vi "PV_Gnl_WaitForViClose.vi"(8 "error in":errorcluster, 10 "TimeOut (ms)":i32, 11 "ViRefNum":refnum<vi>) -> (0 "error out":errorcluster, 3 "ViRefNumDuplicated":refnum<vi>)   [LabVIEW 2020]
doc: "Fonction :\n\nAttend si le VI entré en référence est déchargé de la mémoire, ou si le temps impartit est dépassé.\n\n*****\n\nEntrées :\n\nVIRefNum : référence du VI à vérifier. Dupliquée dans tous les cas. Cette connexion est nécessaire.\n\nTimeOut : temps impartit à cette fonction pour vérifier si le VI est déchargé de la mémoire. Cette connexion est nécessaire.\n\nerror in : entrée d'erreur.\n\n*****\n\nSorties :\n\nVIRefNumDuplicated : référence du VI.\n\nerror out : sortie d'erreur."
panel:
  # "Input"
  # "Output"
  # "Local"
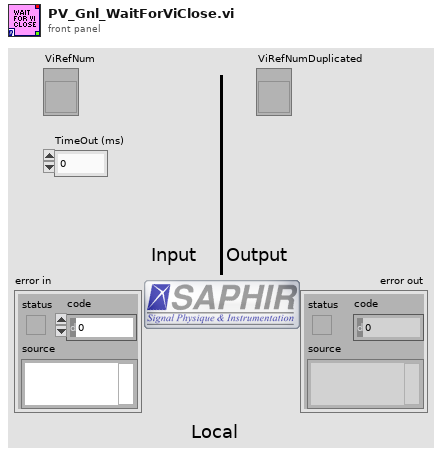
[diagram p1: front panel]
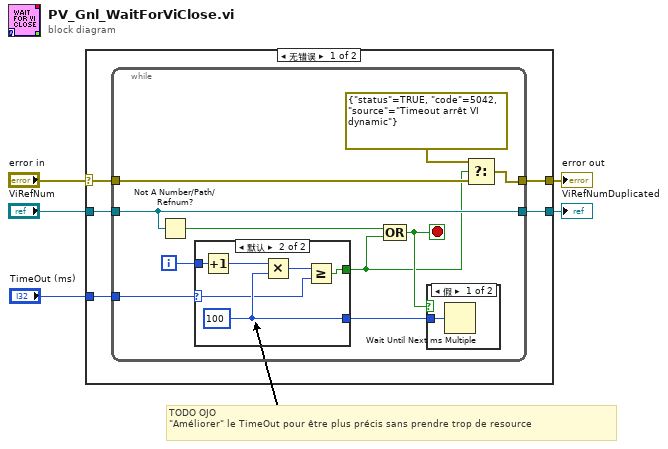
[diagram p0: block diagram]
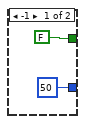
[diagram p2: hidden frame]
diagram:
  # "TODO OJO\n\"Améliorer\" le TimeOut pour être plus précis sans prendre trop de resource"
  n1 = case shown="无错误" "error in" {
    selector: "error in" -> [w9 w31]
    tunnel: [w8 w31] -> w3
    tunnel: "ViRefNum" -> [w10 w30]
    tunnel: [w7 w30] -> w4
    tunnel: "TimeOut (ms)" -> [w6 _]
    frame No Error {
      n2 = while {
        tunnel: w9 -> [w18]
        tunnel: [w20] -> w8
        tunnel: w10 -> [w16]
        tunnel: [w16] -> w7
        tunnel: w6 -> [w13]
        i -> [w14]
        stop <- w15 stop-if-true
        n3 = Not A Number/Path/Refnum?(number/path/refnum=w16) -> (NaN/Path/Refnum?=w17:bool)
        n4 = case shown="默认" w13 {
          selector: w13 -> [_ w23]
          tunnel: w14 -> [_ w25]
          tunnel: [FALSE w28] -> w11
          tunnel: [u32 50 ("millisecond multiple") w27] -> w12
          frame -1 {
          }
          frame Default {
            w27 = 100 ("y")
            n5 = Increment(x=w25) -> (x+1=w26:i32)
            n6 = Multiply(x=w26, y=w27) -> (x*y=w24:i32)
            n7 = Greater Or Equal?(x=w24, y=w23) -> (x >= y?=w28:bool)
          }
        }
        n8 = Compound Arithmetic op=OR(w17, w11) -> (w15:bool)
        n9 = case shown="假" w15 {
          tunnel: w12 -> [w29 _]
          frame False {
            n10 = Wait Until Next ms Multiple(millisecond multiple=w29) -> ()  [unwired: 1 out]
          }
          frame True {
          }
        }
        n11 = Select(t=errorcluster {"status"=TRUE, "code"=5042, "source"="Timeout arrêt VI dynamic"}, s=w11, f=w18) -> (s? t:f=w20:errorcluster)
      }
    }
    frame Error {
    }
  }
  "ViRefNumDuplicated" <- w4
  "error out" <- w3
